vi "Begin.vi"(8 "error in":errorcluster) -> (0 "error out":errorcluster)   [LabVIEW 2016]
doc: "Called before other user functions, this VI is expected to open initial I/O refnums, load in file data, and do all program initialization. Notice that the <B>error out</B> terminal is simply used for data flow. Wiring it to other structures or subVIs ensures that this VI runs first."
uses:
  <vilib>/Rock Robotics/WPI/SafetyOutput/WPI_SafetyOutputConfigMenu.ctl
  <vilib>/Rock Robotics/WPI/DriverStation/WPI_DriverStationRobotMode2.ctl
  <vilib>/Rock Robotics/WPI/Joystick/WPI_JoystickDeviceEnum.ctl
  <vilib>/Rock Robotics/SystemInterfaces/DIO/FPGA_DIOPWMChannel.ctl
  <vilib>/Rock Robotics/SystemInterfaces/DIO/FPGA_DIOChannel.ctl
  <vilib>/Rock Robotics/SystemInterfaces/i2clib/i2c_bus.ctl
  <vilib>/Rock Robotics/SystemInterfaces/DIO/FPGA_DIORelayChannel.ctl
  <vilib>/Rock Robotics/WPI/Relay/WPI_RelayDirection.ctl
  <vilib>/Rock Robotics/WPI/Solenoid/WPI_SolenoidChannel.ctl
  <vilib>/Rock Robotics/WPI/ThirdParty/CanMotor/TalonSRX/WPI_CANTalonSRX_APIControlMode.ctl
  Robot Global Data.vi
  <vilib>/Rock Robotics/Network Tables/NT Write String Array.vi
  <vilib>/Rock Robotics/WPI/MotorControl/WPI_MotorControlOpen VictorSP.vi
  <vilib>/Rock Robotics/WPI/Switch/WPI_SwitchOpenLimit.vi
  <vilib>/Rock Robotics/WPI/RobotDrive/WPI_RobotDriveOpen4MotorWithVictorSP.vi
  <vilib>/Rock Robotics/WPI/Solenoid/WPI_SolenoidOpenSingle.vi
  <vilib>/Rock Robotics/WPI/Counter/WPI_CounterDigitalInputToDigitalSource.vi
  <vilib>/Rock Robotics/WPI/Counter/WPI_CounterOpen UpDown Mode.vi
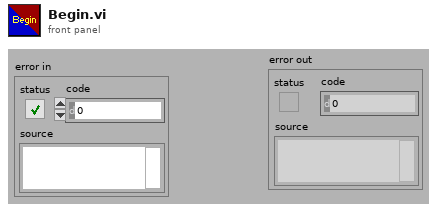
[diagram p1: front panel]
types:
  T1 = typedef "FPGA_DIOChannel.ctl" = enum8{"DIO 0", "DIO 1", "DIO 2", "DIO 3", "DIO 4", "DIO 5", "DIO 6", "DIO 7", "DIO 8", "DIO 9", "DIO MXP 0", "DIO MXP 1", "DIO MXP 2", "DIO MXP 3", "DIO MXP 4", "DIO MXP 5", "DIO MXP 6", "DIO MXP 7", "DIO MXP 8", "DIO MXP 9", "DIO MXP 10", "DIO MXP 11", "DIO MXP 12", "DIO MXP 13", "DIO MXP 14", "DIO MXP 15", "SPI Port CS1", "SPI Port CS2", "SPI Port CS3", "SPI Port MISO", "SPI Port MOSI", "Invalid"}
  T2 = typedef "WPI_SolenoidChannel.ctl" = enum8{"Solenoid 0", "Solenoid 1", "Solenoid 2", "Solenoid 3", "Solenoid 4", "Solenoid 5", "Solenoid 6", "Solenoid 7", "Invalid"}
  T3 = typedef "FPGA_DIOPWMChannel.ctl" = enum8{"PWM 0", "PWM 1", "PWM 2", "PWM 3", "PWM 4", "PWM 5", "PWM 6", "PWM 7", "PWM 8", "PWM 9", "PWM MXP 0", "PWM MXP 1", "PWM MXP 2", "PWM MXP 3", "PWM MXP 4", "PWM MXP 5", "PWM MXP 6", "PWM MXP 7", "PWM MXP 8", "PWM MXP 9", "Invalid"}
  T4 = typedef "WPI_CANTalonSRX_APIControlMode.ctl" = enum8{"Percent VBus", "Speed", "Position", "Slave", "Unchanged / Invalid", "Voltage Compensation", "Current", "Motion Profile", "Motion Magic"}
  T5 = typedef "FPGA_DIORelayChannel.ctl" = enum8{"Relay 0", "Relay 1", "Relay 2", "Relay 3", "Invalid"}
  T6 = typedef "WPI_RelayDirection.ctl" = enum16{"Both directions", "Forward only", "Reverse only"}
  T7 = typedef "i2c_bus.ctl" = enum16{"I2C On-Board", "I2C MXP", "Invalid"}
  T8 = typedef "WPI_JoystickDeviceEnum.ctl" = enum16{"USB 0", "USB 1", "USB 2", "USB 3", "USB 4", "USB 5"}
  T9 = typedef "WPI_DriverStationRobotMode2.ctl" = enum16{"Autonomous Disabled", "Autonomous Enabled", "Teleop Disabled", "Teleop Enabled", "Disconnected", "Finish", "Test Disabled", "Test Enabled", "Emergency Stopped"}
  T10 = typedef "WPI_SafetyOutputConfigMenu.ctl" = enum16{"Enable", "Disable"}
  T11 = typedef "WPI_JoystickDevRef.ctl" = cluster{"Device":T8}
  T12 = typedef "WPI_ServoDeviceRef.ctl" = cluster{"DeviceStatus":errorcluster, "PWM Channel":T3, "DeadBand":T13}
  T13 = typedef "WPI_PWMDeadband.ctl" = cluster{"Name":string, "maxPositivePwm":i32, "minPositivePwm":i32, "centerPwm":i32, "maxNegativePwm":i32, "minNegativePwm":i32, "angularRange":u16}
  T14 = typedef "WPI_MotorControlDeviceRef.ctl" = cluster{"DeviceStatus":errorcluster, "Type":T15, "PWM":cluster{"PWM Channel":T3, "DeadBand":T13}, "CAN":cluster{"Device Number":u8, "SetOutput VI Ref":variant, "GetOutput VI Ref":variant, "Enable VI Ref":variant, "Disable VI Ref":variant, "Data":variant}, "Invert":bool}
  T15 = typedef "WPI_MotorControlType.ctl" = enum16{"PWM", "CAN"}
  T16 = typedef "WPI_RobotDriveDevRef.ctl" = cluster{"DevStatus":errorcluster, "Motors[]":T14[], "Square Inputs":bool, "Max Output":dbl}
  T17 = typedef "WPI_SwitchDevRef.ctl" = cluster{"DevStatus":errorcluster, "DIO Channel":T1, "CntIndex":T18, "Normally Closed":bool}
  T18 = typedef "FPGA_CounterCtrSystemIndex.ctl" = enum8{"Ctr 0", "Ctr 1", "Ctr 2", "Ctr 3", "Ctr 4", "Ctr 5", "Ctr 6", "Ctr 7", "Invalid"}
  T19 = typedef "WPI_I2CDevRef.ctl" = cluster{"DevStatus":errorcluster, "Device Address":u8, "Handle":i32, "I2C Bus":T7}
  T20 = typedef "WPI_RelayDevRef.ctl" = cluster{"DevStatus":errorcluster, "Relay Channel":T5, "Relay Direction":T6}
  T21 = typedef "WPI_SolenoidDevRef.ctl" = cluster{"DevStatus":errorcluster, "Pneumatics Control Module":u8, "Forward Solenoid Channel":T2, "Reverse Solenoid Channel":T2}
  T22 = typedef "WPI_DigitalInputDevRef.ctl" = cluster{"DevStatus":errorcluster, "DIO Channel":T1}
  T23 = typedef "FPGA_CounterEncoderSourceConvertionLVSourceType.ctl" = cluster{"DevStatus":errorcluster, "AnalogTriggerMode?":bool, "DigitalMode":cluster{"DIO Channel":T24}, "AnalogTriggerMode":cluster{"AnalogTriggerIndex":T25, "OutputType":T26}}
  T24 = typedef "FPGA_DIODigitalSourceChannel.ctl" = enum8{"DIO 0", "DIO 1", "DIO 2", "DIO 3", "DIO 4", "DIO 5", "DIO 6", "DIO 7", "DIO 8", "DIO 9", "DIO MXP 0", "DIO MXP 1", "DIO MXP 2", "DIO MXP 3", "DIO MXP 4", "DIO MXP 5", "DIO MXP 6", "DIO MXP 7", "DIO MXP 8", "DIO MXP 9", "DIO MXP 10", "DIO MXP 11", "DIO MXP 12", "DIO MXP 13", "DIO MXP 14", "DIO MXP 15", "Disabled"}
  T25 = typedef "FPGA_AnalogTriggerIndex.ctl" = enum8{"Trig 0", "Trig 1", "Trig 2", "Trig 3", "Trig 4", "Trig 5", "Trig 6", "Trig 7", "Invalid"}
  T26 = typedef "FPGA_AnalogTriggerOutType.ctl" = enum16{"InWindow", "TriggerState", "Rising", "Falling"}
  T27 = typedef "WPI_CounterDevRef.ctl" = cluster{"DevStatus":errorcluster, "CntIndex":T18}
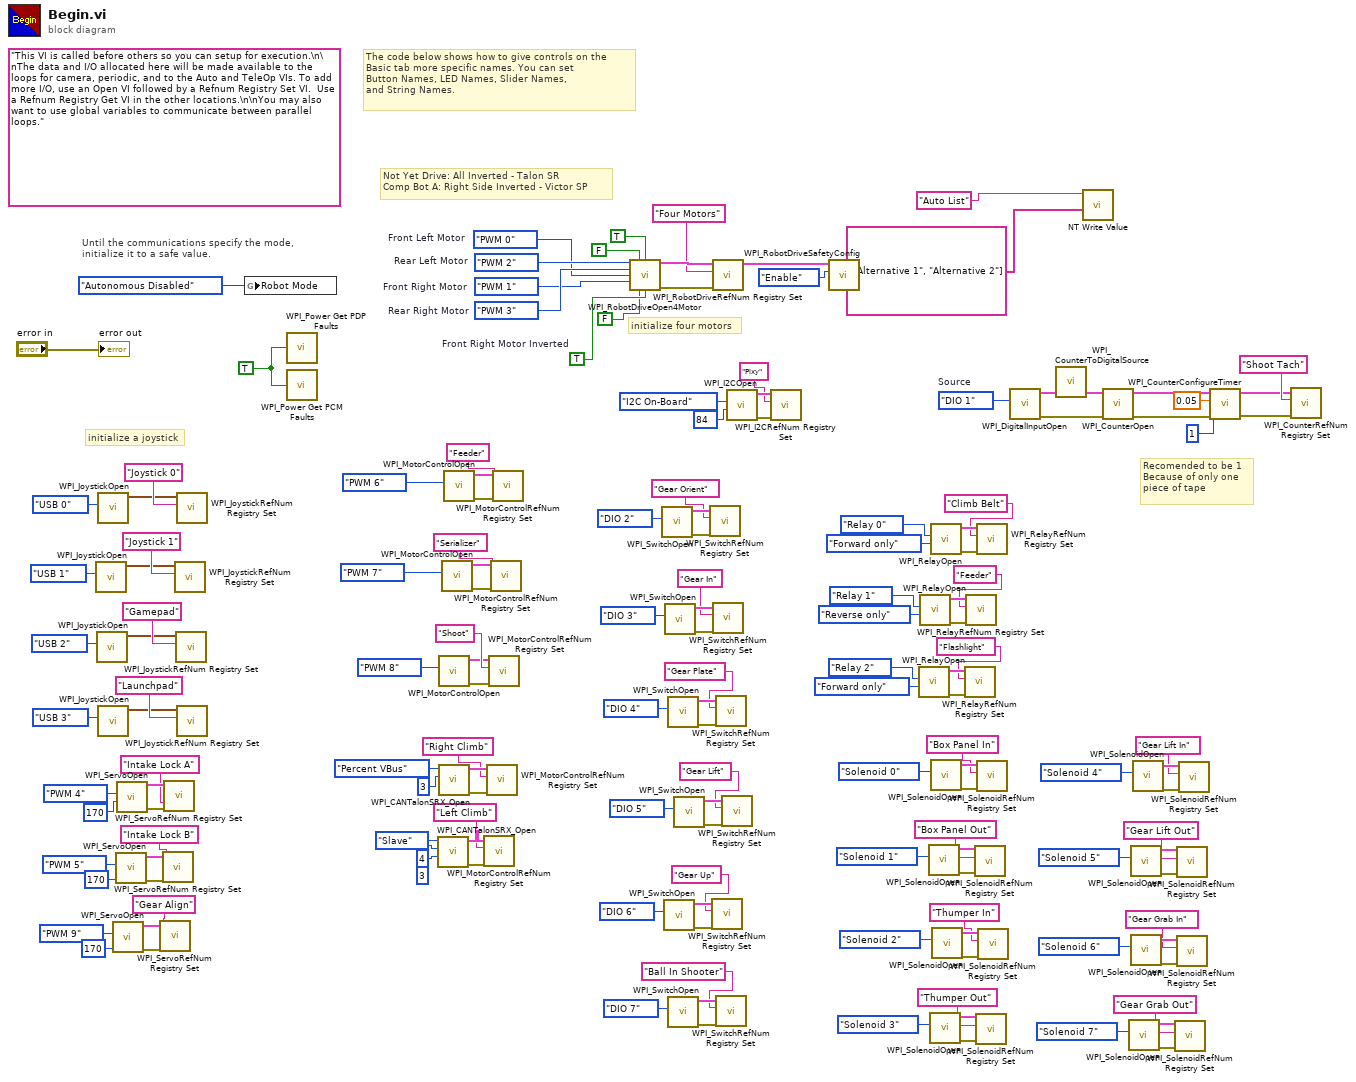
[diagram p0: block diagram]
diagram:
  w10 = FPGA_DIOChannel."DIO 1"  # Source
  w20 = TRUE
  w105 = TRUE  # Front Right Motor Inverted
  w143 = FPGA_DIOPWMChannel."PWM 1"  # Front Right Motor
  w144 = FPGA_DIOPWMChannel."PWM 0"  # Front Left Motor
  w145 = FPGA_DIOPWMChannel."PWM 3"  # Rear Right Motor
  w146 = FPGA_DIOPWMChannel."PWM 2"  # Rear Left Motor
  (unwired) "This VI is called before others so you can setup for execution.\n\nThe data and I/O allocated here will be made available to the loops for camera, periodic, and to the Auto and TeleOp VIs. To add more I/O, use an Open VI followed by a Refnum Registry Set VI.  Use a Refnum Registry Get VI in the other locations.\n\nYou may also want to use global variables to communicate between parallel loops."
  # "Recomended to be 1\nBecause of only one \npiece of tape"
  # "Not Yet Drive: All Inverted - Talon SR\nComp Bot A: Right Side Inverted - Victor SP"
  # "The code below shows how to give controls on the\nBasic tab more specific names. You can set\nButton Names, LED Names, Slider Names,\nand String Names."
  # "initialize a joystick"
  # "Until the communications specify the mode,\ninitialize it to a safe value."
  # "initialize four motors"
  n1 = call <vilib>:"WPI_JoystickOpen.vi"("JoystickDevice"=WPI_JoystickDeviceEnum."USB 1") -> ("JoystickDevRef"=w138:T11)  [unwired: 10 in]
  n2 = call <vilib>:"WPI_JoystickOpen.vi"("JoystickDevice"=WPI_JoystickDeviceEnum."USB 2") -> ("JoystickDevRef"=w135:T11)  [unwired: 10 in]
  n3 = call <vilib>:"WPI_JoystickOpen.vi"("JoystickDevice"=WPI_JoystickDeviceEnum."USB 0") -> ("JoystickDevRef"=w148:T11)  [unwired: 10 in]
  n4 = call <vilib>:"WPI_JoystickOpen.vi"("JoystickDevice"=WPI_JoystickDeviceEnum."USB 3") -> ("JoystickDevRef"=w132:T11)  [unwired: 10 in]
  n5 = call <vilib>:"WPI_ServoOpen.vi"("Angular Range"=u16 170, "PWM Channel"=FPGA_DIOPWMChannel."PWM 9") -> ("error out"=w68:errorcluster, "ServoDeviceRef"=w67:T12)  [unwired: 8 in]
  n6 = call <vilib>:"WPI_ServoOpen.vi"("Angular Range"=u16 170, "PWM Channel"=FPGA_DIOPWMChannel."PWM 5") -> ("error out"=w83:errorcluster, "ServoDeviceRef"=w82:T12)  [unwired: 8 in]
  n7 = call <vilib>:"WPI_ServoOpen.vi"("Angular Range"=u16 170, "PWM Channel"=FPGA_DIOPWMChannel."PWM 4") -> ("error out"=w86:errorcluster, "ServoDeviceRef"=w85:T12)  [unwired: 8 in]
  n8 = call <vilib>:"WPI_ServoRefNum Registry Set.vi"("error in (no error)"=w68, "refnum name"="Gear Align", "ServoDeviceRef"=w67) -> ()  [unwired: 7 in, 2 out]
  n9 = call <vilib>:"WPI_ServoRefNum Registry Set.vi"("error in (no error)"=w83, "refnum name"="Intake Lock B", "ServoDeviceRef"=w82) -> ()  [unwired: 7 in, 2 out]
  n10 = call <vilib>:"WPI_ServoRefNum Registry Set.vi"("error in (no error)"=w86, "refnum name"="Intake Lock A", "ServoDeviceRef"=w85) -> ()  [unwired: 7 in, 2 out]
  n11 = call <vilib>:"WPI_JoystickRefNum Registry Set.vi"("refnum name"="Joystick 1", "JoystickDevRef"=w138) -> ()  [unwired: 8 in, 2 out]
  n12 = call <vilib>:"WPI_JoystickRefNum Registry Set.vi"("refnum name"="Gamepad", "JoystickDevRef"=w135) -> ()  [unwired: 8 in, 2 out]
  n13 = call <vilib>:"WPI_JoystickRefNum Registry Set.vi"("refnum name"="Joystick 0", "JoystickDevRef"=w148) -> ()  [unwired: 8 in, 2 out]
  n14 = call <vilib>:"WPI_JoystickRefNum Registry Set.vi"("refnum name"="Launchpad", "JoystickDevRef"=w132) -> ()  [unwired: 8 in, 2 out]
  n15 = global write "Robot Global Data.vi" "Robot Mode"(WPI_DriverStationRobotMode2."Autonomous Disabled" ("Robot Mode")) -> ()
  n16 = call <vilib>:"WPI_Power Get PDP Faults.vi"("Clear Sticky Faults"=w20) -> ()  [unwired: 10 in, 5 out]
  n17 = call <vilib>:"WPI_Power Get PCM Faults.vi"("Clear Sticky Faults"=w20) -> ()  [unwired: 11 in, 4 out]
  n18 = call <vilib>:"WPI_CANTalonSRX_Open.vi"("Master Device Number"=u8 3, "Device Number"=u8 4, "Control Mode"=WPI_CANTalonSRX_APIControlMode."Slave") -> ("error out"=w61:errorcluster, "CAN Talon SRX Ref"=w60:T14)  [unwired: 7 in]
  n19 = call-poly <vilib>:"WPI_MotorControlOpen.vi"("PWM Channel"=FPGA_DIOPWMChannel."PWM 8") -> ("error out"=w51:errorcluster, "MotorControlDeviceRef"=w50:T14)  [unwired: 9 in]
  n20 = call <vilib>:"WPI_CANTalonSRX_Open.vi"("Device Number"=u8 3, "Control Mode"=WPI_CANTalonSRX_APIControlMode."Percent VBus") -> ("error out"=w63:errorcluster, "CAN Talon SRX Ref"=w62:T14)  [unwired: 8 in]
  n21 = call-poly <vilib>:"WPI_MotorControlOpen.vi"("PWM Channel"=FPGA_DIOPWMChannel."PWM 7") -> ("error out"=w126:errorcluster, "MotorControlDeviceRef"=w125:T14)  [unwired: 9 in]
  n22 = call-poly <vilib>:"WPI_MotorControlOpen.vi"("PWM Channel"=FPGA_DIOPWMChannel."PWM 6") -> ("error out"=w130:errorcluster, "MotorControlDeviceRef"=w129:T14)  [unwired: 9 in]
  n23 = call <vilib>:"WPI_MotorControlRefNum Registry Set.vi"("error in (no error)"=w61, "refnum name"="Left Climb", "MotorControlDevRef"=w60) -> ()  [unwired: 7 in, 2 out]
  n24 = call <vilib>:"WPI_MotorControlRefNum Registry Set.vi"("error in (no error)"=w63, "refnum name"="Right Climb", "MotorControlDevRef"=w62) -> ()  [unwired: 7 in, 2 out]
  n25 = call <vilib>:"WPI_MotorControlRefNum Registry Set.vi"("error in (no error)"=w51, "refnum name"="Shoot", "MotorControlDevRef"=w50) -> ()  [unwired: 7 in, 2 out]
  n26 = call <vilib>:"WPI_MotorControlRefNum Registry Set.vi"("error in (no error)"=w126, "refnum name"="Serializer", "MotorControlDevRef"=w125) -> ()  [unwired: 7 in, 2 out]
  n27 = call <vilib>:"WPI_MotorControlRefNum Registry Set.vi"("error in (no error)"=w130, "refnum name"="Feeder", "MotorControlDevRef"=w129) -> ()  [unwired: 7 in, 2 out]
  n28 = call-poly <vilib>:"WPI_RobotDriveOpen4Motor.vi"("Rear Left Motor"=w146, "Rear Left Motor Inverted"=FALSE, "Rear Right Motor Inverted"=TRUE, "Rear Right Motor"=w145, "Front Left Motor"=w144, "Front Right Motor"=w143, "Front Left Motor Inverted"=FALSE, "Front Right Motor Inverted"=w105) -> ("RobotDriveDevRef"=w155:T16, "error out"=w153:errorcluster)  [unwired: 6 in]
  n29 = call-poly <vilib>:"WPI_SwitchOpen.vi"("DIO Channel"=FPGA_DIOChannel."DIO 2") -> ("error out"=w122:errorcluster, "SwitchDevRef"=w121:T17)  [unwired: 9 in]
  n30 = call-poly <vilib>:"WPI_SwitchOpen.vi"("DIO Channel"=FPGA_DIOChannel."DIO 6") -> ("error out"=w19:errorcluster, "SwitchDevRef"=w18:T17)  [unwired: 9 in]
  n31 = call-poly <vilib>:"WPI_SwitchOpen.vi"("DIO Channel"=FPGA_DIOChannel."DIO 3") -> ("error out"=w118:errorcluster, "SwitchDevRef"=w117:T17)  [unwired: 9 in]
  n32 = call-poly <vilib>:"WPI_SwitchOpen.vi"("DIO Channel"=FPGA_DIOChannel."DIO 4") -> ("error out"=w114:errorcluster, "SwitchDevRef"=w113:T17)  [unwired: 9 in]
  n33 = call-poly <vilib>:"WPI_SwitchOpen.vi"("DIO Channel"=FPGA_DIOChannel."DIO 7") -> ("error out"=w15:errorcluster, "SwitchDevRef"=w14:T17)  [unwired: 9 in]
  n34 = call-poly <vilib>:"WPI_SwitchOpen.vi"("DIO Channel"=FPGA_DIOChannel."DIO 5") -> ("error out"=w24:errorcluster, "SwitchDevRef"=w23:T17)  [unwired: 9 in]
  n35 = call <vilib>:"WPI_SwitchRefNum Registry Set.vi"("error in (no error)"=w122, "refnum name"="Gear Orient", "SwitchDevRef"=w121) -> ()  [unwired: 7 in, 2 out]
  n36 = call <vilib>:"WPI_SwitchRefNum Registry Set.vi"("error in (no error)"=w19, "refnum name"="Gear Up", "SwitchDevRef"=w18) -> ()  [unwired: 7 in, 2 out]
  n37 = call <vilib>:"WPI_RobotDriveRefNum Registry Set.vi"("error in (no error)"=w153, "refnum name"="Four Motors", "RobotDriveDevRef"=w155) -> ("RobotDriveDevRef"=w152:T16)  [unwired: 1 in, 7 out]
  n38 = call <vilib>:"WPI_SwitchRefNum Registry Set.vi"("error in (no error)"=w118, "refnum name"="Gear In", "SwitchDevRef"=w117) -> ()  [unwired: 7 in, 2 out]
  n39 = call <vilib>:"WPI_SwitchRefNum Registry Set.vi"("error in (no error)"=w114, "refnum name"="Gear Plate", "SwitchDevRef"=w113) -> ()  [unwired: 7 in, 2 out]
  n40 = call <vilib>:"WPI_SwitchRefNum Registry Set.vi"("error in (no error)"=w15, "refnum name"="Ball In Shooter", "SwitchDevRef"=w14) -> ()  [unwired: 7 in, 2 out]
  n41 = call <vilib>:"WPI_SwitchRefNum Registry Set.vi"("error in (no error)"=w24, "refnum name"="Gear Lift", "SwitchDevRef"=w23) -> ()  [unwired: 7 in, 2 out]
  n42 = call <vilib>:"WPI_I2COpen.vi"("Device Address"=u8 84, "I2C Bus"=i2c_bus."I2C On-Board") -> ("error out"=w110:errorcluster, "I2CDevRef"=w109:T19)  [unwired: 8 in]
  n43 = call <vilib>:"WPI_I2CRefNum Registry Set.vi"("error in (no error)"=w110, "refnum name"="Pixy", "I2CDevRef"=w109) -> ()  [unwired: 7 in, 2 out]
  n44 = call <vilib>:"WPI_RobotDriveSafetyConfig.vi"("mode"=WPI_SafetyOutputConfigMenu."Enable", "RobotDriveDevRef"=w152) -> ()  [unwired: 8 in, 2 out]
  n45 = call <vilib>:"WPI_RelayOpen.vi"("Relay Direction"=WPI_RelayDirection."Forward only", "Relay Channel"=FPGA_DIORelayChannel."Relay 2") -> ("error out"=w101:errorcluster, "RelayDevRef"=w100:T20)  [unwired: 8 in]
  n46 = call <vilib>:"WPI_RelayOpen.vi"("Relay Direction"=WPI_RelayDirection."Reverse only", "Relay Channel"=FPGA_DIORelayChannel."Relay 1") -> ("error out"=w91:errorcluster, "RelayDevRef"=w90:T20)  [unwired: 8 in]
  n47 = call-poly <vilib>:"WPI_SolenoidOpen.vi"("Solenoid Channel"=WPI_SolenoidChannel."Solenoid 1") -> ("error out"=w72:errorcluster, "SolenoidDevRef"=w71:T21)  [unwired: 9 in]
  n48 = call-poly <vilib>:"WPI_SolenoidOpen.vi"("Solenoid Channel"=WPI_SolenoidChannel."Solenoid 3") -> ("error out"=w44:errorcluster, "SolenoidDevRef"=w43:T21)  [unwired: 9 in]
  n49 = call <vilib>:"WPI_RelayOpen.vi"("Relay Direction"=WPI_RelayDirection."Forward only", "Relay Channel"=FPGA_DIORelayChannel."Relay 0") -> ("error out"=w96:errorcluster, "RelayDevRef"=w95:T20)  [unwired: 8 in]
  n50 = call-poly <vilib>:"WPI_SolenoidOpen.vi"("Solenoid Channel"=WPI_SolenoidChannel."Solenoid 0") -> ("error out"=w76:errorcluster, "SolenoidDevRef"=w75:T21)  [unwired: 9 in]
  n51 = call-poly <vilib>:"WPI_SolenoidOpen.vi"("Solenoid Channel"=WPI_SolenoidChannel."Solenoid 2") -> ("error out"=w48:errorcluster, "SolenoidDevRef"=w47:T21)  [unwired: 9 in]
  n52 = call <vilib>:"WPI_RelayRefNum Registry Set.vi"("error in (no error)"=w101, "refnum name"="Flashlight", "RelayDevRef"=w100) -> ()  [unwired: 7 in, 2 out]
  n53 = call <vilib>:"WPI_RelayRefNum Registry Set.vi"("error in (no error)"=w91, "refnum name"="Feeder", "RelayDevRef"=w90) -> ()  [unwired: 7 in, 2 out]
  n54 = call <vilib>:"WPI_SolenoidRefNum Registry Set.vi"("error in (no error)"=w72, "refnum name"="Box Panel Out", "SolenoidDevRef"=w71) -> ()  [unwired: 7 in, 2 out]
  n55 = call <vilib>:"WPI_SolenoidRefNum Registry Set.vi"("error in (no error)"=w44, "refnum name"="Thumper Out", "SolenoidDevRef"=w43) -> ()  [unwired: 7 in, 2 out]
  n56 = call <vilib>:"WPI_RelayRefNum Registry Set.vi"("error in (no error)"=w96, "refnum name"="Climb Belt", "RelayDevRef"=w95) -> ()  [unwired: 7 in, 2 out]
  n57 = call <vilib>:"WPI_SolenoidRefNum Registry Set.vi"("error in (no error)"=w76, "refnum name"="Box Panel In", "SolenoidDevRef"=w75) -> ()  [unwired: 7 in, 2 out]
  n58 = call <vilib>:"WPI_SolenoidRefNum Registry Set.vi"("error in (no error)"=w48, "refnum name"="Thumper In", "SolenoidDevRef"=w47) -> ()  [unwired: 7 in, 2 out]
  n59 = call <vilib>:"WPI_DigitalInputOpen.vi"("DIO Channel"=w10) -> ("error out"=w5:errorcluster, "DigitalInputDevRef"=w9:T22)  [unwired: 1 in, 8 out]
  n60 = call-poly <vilib>:"WPI_CounterToDigitalSource.vi"("DigitalInputDevRef"=w9) -> ("Digital Source"=w11:T23)  [unwired: 6 out]
  n61 = call-poly <vilib>:"NT Write Value.vi"("String Array"=string[] ["Alternative 1", "Alternative 2"], "Name"="Auto List") -> ()  [unwired: 9 in, 1 out]
  n62 = call-poly <vilib>:"WPI_CounterOpen.vi"("error in (no error)"=w5, "Up Source"=w11) -> ("error out"=w7:errorcluster, "CounterDevRef"=w6:T27)  [unwired: 5 in, 3 out]
  n63 = call-poly <vilib>:"WPI_SolenoidOpen.vi"("Solenoid Channel"=WPI_SolenoidChannel."Solenoid 7") -> ("error out"=w28:errorcluster, "SolenoidDevRef"=w27:T21)  [unwired: 9 in]
  n64 = call-poly <vilib>:"WPI_SolenoidOpen.vi"("Solenoid Channel"=WPI_SolenoidChannel."Solenoid 5") -> ("error out"=w36:errorcluster, "SolenoidDevRef"=w35:T21)  [unwired: 9 in]
  n65 = call-poly <vilib>:"WPI_SolenoidOpen.vi"("Solenoid Channel"=WPI_SolenoidChannel."Solenoid 6") -> ("error out"=w32:errorcluster, "SolenoidDevRef"=w31:T21)  [unwired: 9 in]
  n66 = call-poly <vilib>:"WPI_SolenoidOpen.vi"("Solenoid Channel"=WPI_SolenoidChannel."Solenoid 4") -> ("error out"=w40:errorcluster, "SolenoidDevRef"=w39:T21)  [unwired: 9 in]
  n67 = call <vilib>:"WPI_SolenoidRefNum Registry Set.vi"("error in (no error)"=w28, "refnum name"="Gear Grab Out", "SolenoidDevRef"=w27) -> ()  [unwired: 7 in, 2 out]
  n68 = call <vilib>:"WPI_SolenoidRefNum Registry Set.vi"("error in (no error)"=w36, "refnum name"="Gear Lift Out", "SolenoidDevRef"=w35) -> ()  [unwired: 7 in, 2 out]
  n69 = call <vilib>:"WPI_SolenoidRefNum Registry Set.vi"("error in (no error)"=w32, "refnum name"="Gear Grab In", "SolenoidDevRef"=w31) -> ()  [unwired: 7 in, 2 out]
  n70 = call <vilib>:"WPI_SolenoidRefNum Registry Set.vi"("error in (no error)"=w40, "refnum name"="Gear Lift In", "SolenoidDevRef"=w39) -> ()  [unwired: 7 in, 2 out]
  n71 = call <vilib>:"WPI_CounterConfigureTimer.vi"("error in (no error)"=w7, "Number Samples to Average"=u8 1, "MaxPeriod (sec)"=0.05, "CounterDevRef in"=w6) -> ("error out"=w1:errorcluster, "CounterDevRef out"=w2:T27)  [unwired: 6 in]
  n72 = call <vilib>:"WPI_CounterRefNum Registry Set.vi"("error in (no error)"=w1, "refnum name"="Shoot Tach", "CounterDevRef"=w2) -> ()  [unwired: 7 in, 2 out]
  "error out" <- "error in"
